vi "PPMS Monitor and Control.vi"(8 "Refresh Rate":dbl=1.346, 11 "IP Address":string="130.49.180.72") -> (1 "Field (Oe)":dbl=-0.00879339873790741, 3 "Temperature(K)":dbl=147.5612 format="%#_5g")   [LabVIEW 2013]
doc: "This VI monitors the PPMS temperature and magnetic field using QD Labview interface. These values are continuously updated to a global variable."
uses:
  PPMS Global.vi
panel:
  in  "Temp Approach":i32(ring) items=["FastSettle", "NoOvershoot"]
  in  "CC - Optional":string
  in  "Recipient's Email Address":string
  in  "Low Helium Level Notify?":bool
  in  "Helium Notification Level":dbl=1.0
  out "Helium Level":dbl=79.9
  out "Position":dbl=90.002
  out "Temperature Status":i32(ring)=10 items=["TemperatureUnknown"=0, "Stable"=1, "Tracking"=2, "Near"=5, "Chasing"=6, "Filling"=7, "Standby"=10, "Disabled"=13, "ImpedanceNotFunction"=14, "TempFailure"=15]
  # "Do not close!       Keep this VI running at all times!"
  # "This VI will not respond to set-field requests if target field is  larger than ±5T, or if helium level is below 70%"
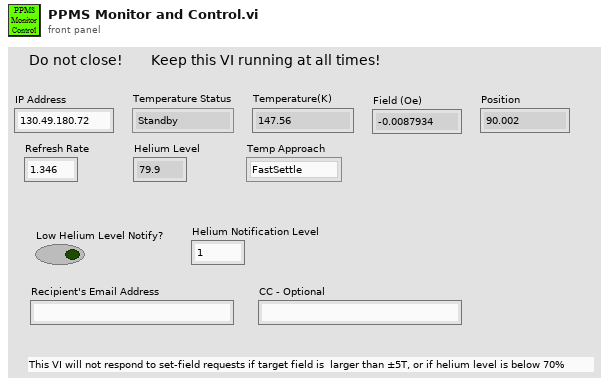
[diagram p1: front panel]
types:
  T1 = enum16{"0", "1", "2", "3", "4", "5", "6", "7", "8", "9", "10", "11", "12", "13", "14"}
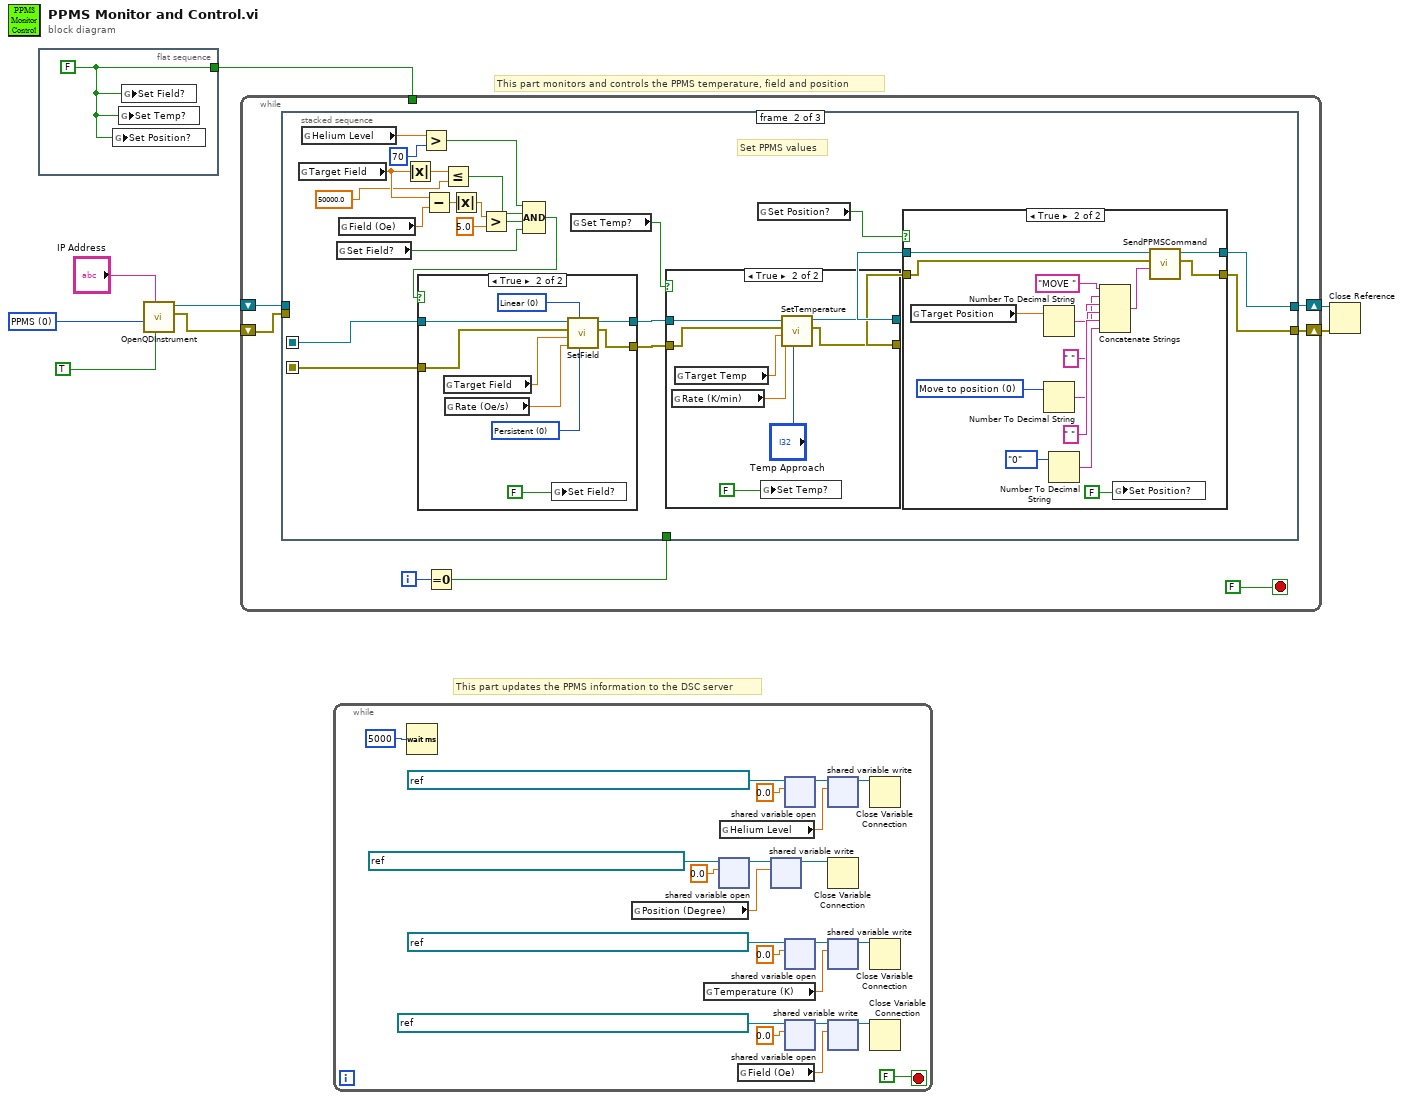
[diagram p0: block diagram]
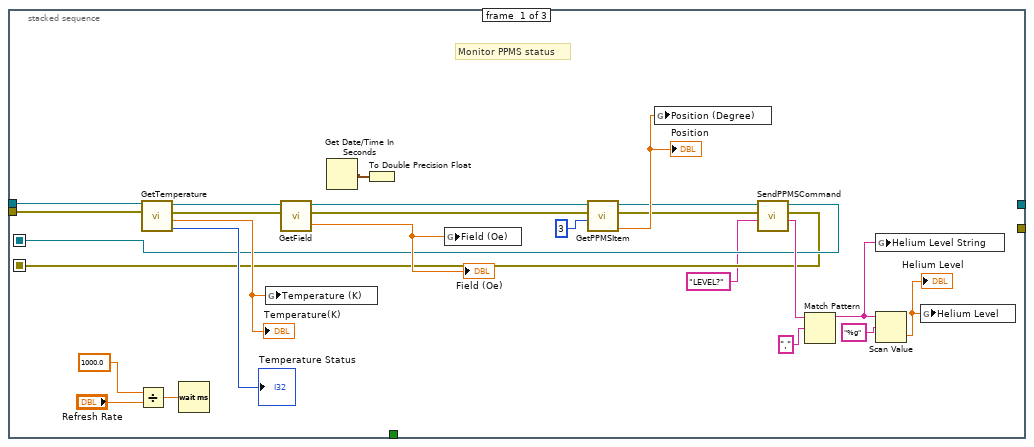
[diagram p2: hidden frame]
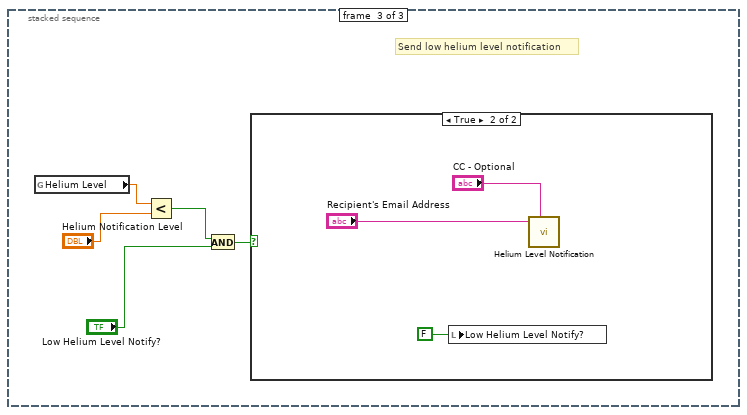
[diagram p6: hidden frame]
diagram:
  w6 = 0 items=["PPMS", "VersaLab", "DynaCool", "SVSM"] ("Instrument\nType")
  # "This part updates the PPMS information to the DSC server"
  # "This part monitors and controls the PPMS temperature, field and position"
  n1 = flat-sequence {
    tunnel: [w9] -> w3
    frame #0 {
      w9 = FALSE ("Set Field?")
      n2 = global write "PPMS Global.vi" "Set Position?"(w9) -> ()
      n3 = global write "PPMS Global.vi" "Set Temp?"(w9) -> ()
      n4 = global write "PPMS Global.vi" "Set Field?"(w9) -> ()
    }
  }
  n5 = call "OpenQDInstrument.vi"("Remote"=TRUE, "IP Address"="IP Address", "Instrument Type"=w6) -> ("error out"=w4:errorcluster, "Instrument Ref"=w5:refnum<k24>)  [unwired: 5 in]
  n6 = while {
    tunnel: w3 -> [_]
    shift-right: [w12] -> w2
    shift-left: w5 -> [w16]
    shift-right: [w11] -> w1
    shift-left: w4 -> [w15]
    i -> [w14]
    stop <- FALSE stop-if-true
    n7 = Equal To 0?(x=w14) -> (x = 0?=w13:bool)
    n8 = stacked-sequence {
      seq-local: [w21 _ _] -> [_ w63 _]
      seq-local: [w20 _ _] -> [_ w62 _]
      tunnel: w16 -> [w41 _ _]
      tunnel: w15 -> [w40 _ _]
      tunnel: w13 -> [_ _ _]
      tunnel: [_ w53 _] -> w12
      tunnel: [_ w52 _] -> w11
      frame #0 {
        # "Monitor PPMS status"
        n9 = Divide(x=1000.0 ("milliseconds to wait"), y="Refresh Rate") -> (x/y=w27:dbl)
        n10 = call "GetTemperature.vi"("error in (no error)"=w40, "Instrument Ref In"=w41) -> ("Temperature\nStatus"=→"Temperature Status":i32, "Temperature"=w34:dbl, "error out"=w37:errorcluster, "Instrument Ref Out"=w36:refnum<k24>)  [unwired: 3 in, 1 out]
        "Temperature(K)" <- w34
        n11 = Wait (ms)(milliseconds to wait=w27) -> ()  [unwired: 1 out]
        n12 = global write "PPMS Global.vi" "Temperature (K)"(w34) -> ()
        n13 = call "GetField.vi"("error in (no error)"=w37, "Instrument Ref In"=w36) -> ("Field"=w35:dbl, "error out"=w31:errorcluster, "Instrument Ref Out"=w32:refnum<k24>)  [unwired: 3 in, 2 out]
        "Field (Oe)" <- w35
        n14 = Get Date/Time In Seconds() -> (seconds since 1Jan1904=w38:timestamp)
        n15 = To Double Precision Float(number=w38) -> ()  [unwired: 1 out]
        n16 = global write "PPMS Global.vi" "Field (Oe)"(w35) -> ()
        n17 = call "GetPPMSItem.vi"("Channel"=3, "error in (no error)"=w31, "Instrument Ref In"=w32) -> ("Result"=w30:dbl, "error out"=w22:errorcluster, "Instrument Ref Out"=w23:refnum<k24>)  [unwired: 1 in, 1 out]
        "Position" <- w30
        n18 = global write "PPMS Global.vi" "Position (Degree)"(w30) -> ()
        n19 = call "SendPPMSCommand.vi"("PpmsCommand"="LEVEL?", "error in (no error)"=w22, "Instrument Ref In"=w23) -> ("PpmsReply"=w24:string, "error out"=w20:errorcluster, "Instrument Ref Out"=w21:refnum<k24>)  [unwired: 4 in, 2 out]
        n20 = Match Pattern(string=w24, regular expression=",") -> (before substring=w17:string)  [unwired: 1 in, 3 out]
        n21 = global write "PPMS Global.vi" "Helium Level String"(w17) -> ()
        n22 = Scan Value(string=w17, format string="%g") -> (value=w18:dbl)  [unwired: 1 in, 1 out]
        "Helium Level" <- w18
        n23 = global write "PPMS Global.vi" "Helium Level"(w18) -> ()
      }
      frame #1 {
        # "Set PPMS values"
        n24 = global read "PPMS Global.vi" "Target Field"() -> (w51:dbl)
        n25 = global read "PPMS Global.vi" "Helium Level"() -> (w44:dbl)
        n26 = global read "PPMS Global.vi" "Set Field?"() -> (w46:bool)
        n27 = global read "PPMS Global.vi" "Field (Oe)"() -> (w57:dbl)
        n28 = Absolute Value(x=w51) -> (abs(x)=w50:dbl)
        n29 = Greater?(x=w44, y=70) -> (0:w42:bool)
        n30 = Subtract(x=w51, y=w57) -> (x-y=w56:dbl)
        n31 = Less Or Equal?(x=w50, y=50000.0) -> (x <= y?=w47:bool)
        n32 = Absolute Value(x=w56) -> (abs(x)=w55:dbl)
        n33 = Greater?(x=w55, y=5.0) -> (0:w48:bool)
        n34 = Compound Arithmetic op=AND(w42, w47, w48, w46) -> (w45:bool)
        n35 = case shown="True" w45 {
          tunnel: w63 -> [w94 w101]
          tunnel: w62 -> [w93 w100]
          tunnel: [w94 w97] -> w61
          tunnel: [w93 w96] -> w60
          frame False {
          }
          frame True {
            w102 = 0 items=["Linear", "NoOvershoot", "Oscillate"] ("Approach")
            w103 = 0 items=["Persistent", "Driven"] ("Mode")
            n36 = global read "PPMS Global.vi" "Target Field"() -> (w99:dbl)
            n37 = global read "PPMS Global.vi" "Rate (Oe/s)"() -> (w98:dbl)
            n38 = global write "PPMS Global.vi" "Set Field?"(FALSE ("Set Field?")) -> ()
            n39 = call "SetField.vi"("Mode"=w103, "Approach"=w102, "Rate"=w98, "Field"=w99, "error in (no error)"=w100, "Instrument Ref In"=w101) -> ("error out"=w96:errorcluster, "Instrument Ref Out"=w97:refnum<k24>)  [unwired: 1 in, 1 out]
          }
        }
        n40 = global read "PPMS Global.vi" "Set Temp?"() -> (w65:bool)
        n41 = case shown="True" w65 {
          tunnel: w61 -> [w84 w91]
          tunnel: w60 -> [w83 w90]
          tunnel: [w84 w87] -> w59
          tunnel: [w83 w86] -> w58
          frame False {
          }
          frame True {
            n42 = global read "PPMS Global.vi" "Rate (K/min)"() -> (w88:dbl)
            n43 = global read "PPMS Global.vi" "Target Temp"() -> (w89:dbl)
            n44 = global write "PPMS Global.vi" "Set Temp?"(FALSE ("Set Field?")) -> ()
            n45 = call "SetTemperature.vi"("Approach"="Temp Approach", "Rate"=w88, "Temperature"=w89, "error in (no error)"=w90, "Instrument Ref In"=w91) -> ("error out"=w86:errorcluster, "Instrument Ref Out"=w87:refnum<k24>)  [unwired: 2 in, 1 out]
          }
        }
        n46 = global read "PPMS Global.vi" "Set Position?"() -> (w64:bool)
        n47 = case shown="True" w64 {
          tunnel: w59 -> [w67 w72]
          tunnel: w58 -> [w66 w71]
          tunnel: [w67 w70] -> w53
          tunnel: [w66 w69] -> w52
          frame False {
          }
          frame True {
            w77 = u16 0 items=["Move to position", "Move to limit", "Redefine current position", ""] ("Mode")
            n48 = global read "PPMS Global.vi" "Target Position"() -> (w73:dbl)
            n49 = Number To Decimal String(number=w73) -> (decimal integer string=w75:string)  [unwired: 1 in]
            n50 = Number To Decimal String(number=w77) -> (decimal integer string=w78:string)  [unwired: 1 in]
            n51 = Number To Decimal String(number=T1."0" ("Slow down code\ndefault = 0")) -> (decimal integer string=w81:string)  [unwired: 1 in]
            n52 = Concatenate Strings("MOVE " ("string"), w75, " " ("string"), w78, " " ("string"), w81) -> (w82:string)
            n53 = global write "PPMS Global.vi" "Set Position?"(FALSE ("Set Field?")) -> ()
            n54 = call "SendPPMSCommand.vi"("PpmsCommand"=w82, "error in (no error)"=w71, "Instrument Ref In"=w72) -> ("error out"=w69:errorcluster, "Instrument Ref Out"=w70:refnum<k24>)  [unwired: 4 in, 3 out]
          }
        }
      }
      frame #2 {
        # "Send low helium level notification"
        n55 = global read "PPMS Global.vi" "Helium Level"() -> (w108:dbl)
        n56 = Less?(x=w108, y="Helium Notification Level") -> (x < y?=w104:bool)
        n57 = And(x=w104, y="Low Helium Level Notify?") -> (x .and. y?=w106:bool)
        n58 = case shown="True" w106 {
          frame False {
          }
          frame True {
            n59 = local write "Low Helium Level Notify?"(FALSE ("Low Helium Level Notify?")) -> ()
            n60 = call "Helium Level Notification.vi"("Recipient's Email Address"="Recipient's Email Address", "CC - Optional"="CC - Optional") -> ()  [unwired: 4 in]
          }
        }
      }
    }
  }
  n61 = while {
    stop <- FALSE stop-if-true
    n62 = Wait (ms)(milliseconds to wait=u32 5000) -> ()  [unwired: 1 out]
    n63 = global read "PPMS Global.vi" "Position (Degree)"() -> (w114:dbl)
    n64 = global read "PPMS Global.vi" "Temperature (K)"() -> (w124:dbl)
    n65 = shared-variable-open(refnum<k21> "ni.var.psp://housesoftheholy/PPMS 2/PPMS 2 Position" ("shared variable refnum in"), 0.0) -> (w118:refnum<k21>)  [unwired: 2 in, 1 out]
    n66 = global read "PPMS Global.vi" "Helium Level"() -> (w119:dbl)
    n67 = global read "PPMS Global.vi" "Field (Oe)"() -> (w132:dbl)
    n68 = shared-variable-write(w118, w114) -> (w117:refnum<k21>)  [unwired: 1 in, 1 out]
    n69 = shared-variable-open(refnum<k21> "ni.var.psp://housesoftheholy/PPMS 2/PPMS 2 Helium Level" ("shared variable refnum in"), 0.0) -> (w123:refnum<k21>)  [unwired: 2 in, 1 out]
    n70 = shared-variable-open(refnum<k21> "ni.var.psp://housesoftheholy/PPMS 2/PPMS 2 Temperature" ("shared variable refnum in"), 0.0) -> (w128:refnum<k21>)  [unwired: 2 in, 1 out]
    n71 = shared-variable-open(refnum<k21> "ni.var.psp://housesoftheholy/PPMS 2/PPMS 2 Magnetic Field" ("shared variable refnum in"), 0.0) -> (w131:refnum<k21>)  [unwired: 2 in, 1 out]
    n72 = shared-variable-write(w123, w119) -> (w122:refnum<k21>)  [unwired: 1 in, 1 out]
    n73 = Close Variable Connection(11:w117) -> ()  [unwired: 1 in, 1 out]
    n74 = shared-variable-write(w128, w124) -> (w127:refnum<k21>)  [unwired: 1 in, 1 out]
    n75 = shared-variable-write(w131, w132) -> (w130:refnum<k21>)  [unwired: 1 in, 1 out]
    n76 = Close Variable Connection(11:w122) -> ()  [unwired: 1 in, 1 out]
    n77 = Close Variable Connection(11:w127) -> ()  [unwired: 1 in, 1 out]
    n78 = Close Variable Connection(11:w130) -> ()  [unwired: 1 in, 1 out]
  }
  n79 = Close Reference(reference=w2, error in (no error)=w1) -> ()  [unwired: 1 out]
